vi "Play Path.vi"(4 "Align for Path":bool, 6 "Synchronication":enum16{"Start", "Wait"}(ring), 7 "Description":string, 8 "Command Info In":T1, 9 "Reverse (T) / Normal (F)":bool, 10 "Path Reversed":bool, 11 "Path":path) -> (0 "Command Info Out":T1)   [LabVIEW 2019]
doc: "This VI notifies the subsystem to the new setpoint."
uses:
  <vilib>/Rock Robotics/WPI/Framework/Command Status Info.ctl
  <vilib>/Rock Robotics/WPI/Framework/Completion Status.ctl
  <vilib>/Rock Robotics/WPI/Framework/Completion Notifier.ctl
  Implementation/Drive Setpoints.ctl
  Implementation/Drive Operations.ctl
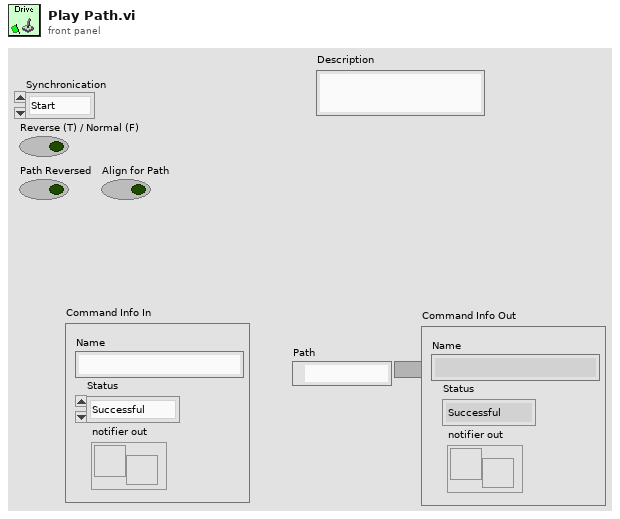
[diagram p1: front panel]
types:
  T1 = typedef "Command Status Info.ctl" = cluster{"Name":string, "Status":T2, "notifier out":T3}
  T2 = typedef "Completion Status.ctl" = enum16{"Successful", "Aborted", "Incomplete"}
  T3 = typedef "Completion Notifier.ctl" = refnum<notifier>
  T4 = typedef "Drive Operations.ctl" = enum16{"Reserve", "Read Current", "Immediate", "Drive for Time", "Drive for Distance", "Play Path"}
  T5 = cluster{"V":dbl[], "Theta":dbl[], "Sample Period":dbl}
  T6 = typedef "Drive Setpoints.ctl" = cluster{"Operation":T4, "Left Setpoint":dbl, "Right Setpoint":dbl, "Auto Path Data":cluster{"V":dbl[], "Theta":dbl[], "Sample Period":dbl}}
  T7 = cluster{"Segment Name":string, "Type":enum16{"Accel Straight", "Const Straight", "Blend", "Circle"}, "Traj Pos Points":cluster{"x":dbl, "y":dbl, "th":dbl}[], "Traj Vel Points":cluster{"V":dbl, "th":dbl}[], "Accel Index":i32, "Decel Index":i32}[]
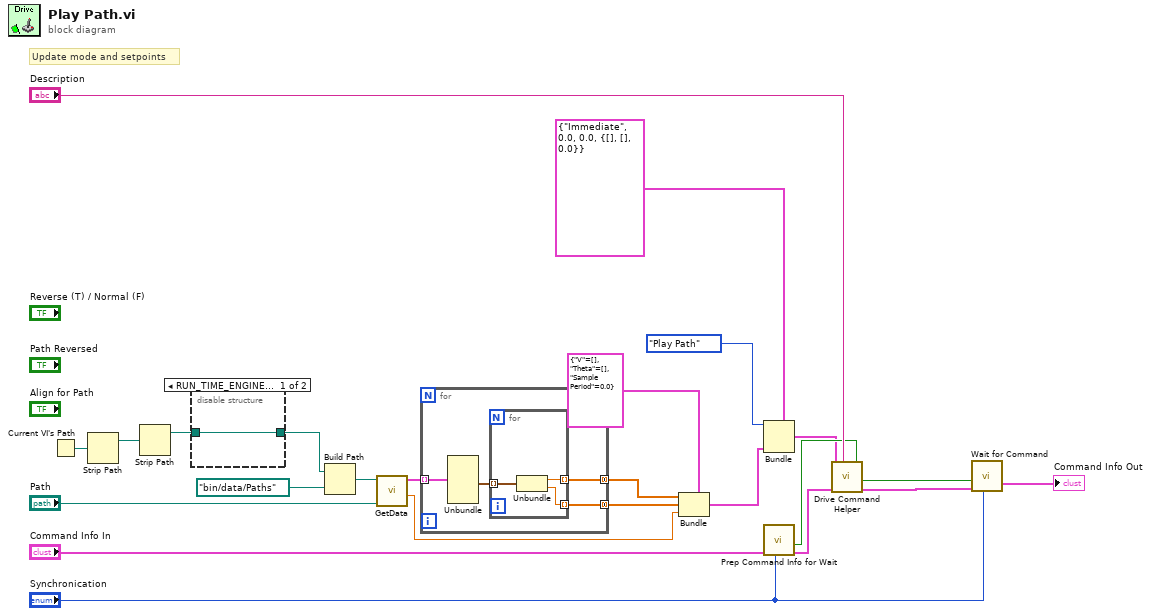
[diagram p0: block diagram]
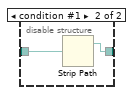
[diagram p2: hidden frame]
diagram:
  # "Update mode and setpoints"
  n1 = Current VI's Path() -> (path=w13:path)
  n2 = Strip Path(path=w13) -> (stripped path=w12:path)  [unwired: 1 out]
  n3 = Strip Path(path=w12) -> (stripped path=w9:path)  [unwired: 1 out]
  n4 = disable-structure shown="RUN_TIME_ENGINE==False" {
    disable-tunnel: [w24 w25] -> w10
    disable-tunnel: w9 -> [w24 w26]
    frame condition #0 (active) {
    }
    frame condition #1 {
      n5 = Strip Path(path=w26) -> (stripped path=w25:path)  [unwired: 1 out]
    }
  }
  n6 = Build Path(base path=w10, name or relative path=path "bin/data/Paths") -> (appended path=w14:path)
  n7 = call "GetData.vi"("File"="Path", "file (use dialog)"=w14) -> ("Sample Period (s)"=w2:dbl, "Trajectory Data"=w15:T7)  [unwired: 2 in, 6 out]
  n8 = for {
    tunnel: [w30] -> w8 mode=concatenating
    tunnel: [w29] -> w7 mode=concatenating
    tunnel: w15 -> [w27] mode=indexing
    n9 = Unbundle(w27) -> ("Traj Vel Points"=w28:cluster{"V":dbl, "th":dbl}[])  [unwired: 5 out]
    n10 = for {
      tunnel: w28 -> [w31] mode=indexing
      tunnel: [w33] -> w30 mode=indexing
      tunnel: [w32] -> w29 mode=indexing
      n11 = Unbundle(w31) -> ("V"=w33:dbl, "th"=w32:dbl)
    }
  }
  n12 = Bundle(cluster=T5 {"V"=[], "Theta"=[], "Sample Period"=0.0} ("Auto Path Data"), "V"=w8, "Theta"=w7, "Sample Period"=w2) -> (w1:T5)
  n13 = Bundle(cluster=T6 {"Operation"=enum."Immediate", "Left Setpoint"=0.0, "Right Setpoint"=0.0, "Auto Path Data"={"V"=[], "Theta"=[], "Sample Period"=0.0}} ("SubSystem Data"), "Operation"=Drive_Operations."Play Path", "Auto Path Data"=w1) -> (w3:T6)  [unwired: 2 in]
  n14 = call <vilib>:"Prep Command Info for Wait.vi"("Synchronication"="Synchronication", "Command Info"="Command Info In") -> ("Command Info"=w21:T1, "Allocated"=w17:bool)  [unwired: 8 in]
  n15 = call "Drive Command Helper.vi"("Description"="Description", "Command Info In"=w21, "SubSystem Data"=w3) -> ("Command Info Out"=w20:T1)  [unwired: 6 in, 2 out]
  n16 = call <vilib>:"Wait for Command.vi"("Synchronication"="Synchronication", "Command Info in"=w20, "Allocated"=w17) -> ("Command Info out"=→"Command Info Out":T1)  [unwired: 8 in]
